vi "TestCSCom.vi"() -> ()   [LabVIEW 2017]
uses:
  C:/Code/CMCryoSysCode/LVPort/CSCom/bin/Debug/CSCom.dll
  CSCom/bin/Debug/CSCom.dll
panel:
  in  "Data to send":T1
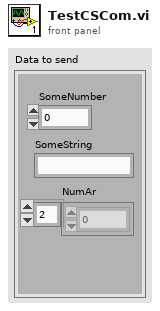
[diagram p1: front panel]
types:
  T1 = cluster{"SomeNumber":dbl, "SomeString":string, "NumAr":dbl[]}
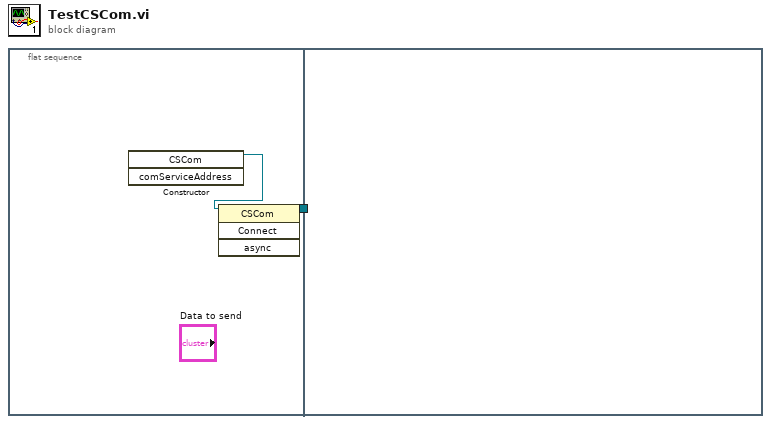
[diagram p0: block diagram]
diagram:
  n1 = flat-sequence {
    tunnel: [w2] -> w1
    tunnel: w1 -> [_]
    frame #0 {
      n2 = constructor class="CSCom"() -> (reference out=w3:refnum<k24>)  [unwired: 4 in, 3 out]
      n3 = invoke class="CSCom" method="Connect"(reference=w3) -> (reference out=w2:refnum<k24>)  [unwired: 3 in, 3 out]
    }
    frame #1 {
    }
  }
